vi "Unibot.vi"() -> ()   [LabVIEW 2012]
doc: "Pendubot (Pendulum Robot) consists of a DC motor connected to a link physical rigid link (called here 'elbow\") which is connected to a second rigid link ('arm\") that has no actuation (free spinning link).\n\nThe control objective is to keep the free link in the vertical position while you can choose to balance the controller link (called here elbow) in the extended position (both links are up) or in the contracted position (elbow pointing down and free link up). In those operating points, a State Feedback Control is used to keep in Up-Up or Down-Up position.\n\nThis VI demonstrates how to use Linearization, design of LQR and pole placement controllers and use on swiching controller."
uses:
  <vilib>/Simulation/Scripting/Companion Diagram/SimConfigNode/SimDog.xnode
  <vilib>/Simulation/SignalDisplay/Implementation/NILVSim Time Waveform.llb/SIM Time Waveform (scalar).vi
  <vilib>/Simulation/Implementation/Shared/SIMSCR Execution Mode.ctl
  <vilib>/addons/Control Design/_State Feedback Control/NI_CD_State Feedback Control.lvlib
  <vilib>/addons/Control Design/_Utility/NI_CD_Model Viewer.lvlib
  <vilib>/Simulation/Utility/Implementation/SIM Halt.vi
  Control Systems/Non-linear/Unibot - State Machine Controller.vi
  <vilib>/addons/Control Design/_State Feedback Control/State Feedback Control.llb/State Feedback Control SubVis/cd_Discretized Linear Quadratic Regulator.vi
  <vilib>/Simulation/Scripting/Companion Diagram/SimConfigNode/_simSolvers.ctl
  <vilib>/Simulation/Scripting/Companion Diagram/SimConfigNode/SimParams.ctl
  <vilib>/addons/Control Design/_Model Reduction/NI_CD_Model Reduction.lvlib
  <vilib>/addons/Control Design/_Time Response Analysis/NI_CD_Time Response.lvlib
  <vilib>/addons/Control Design/_Utility/NI_LinSys_Polynomial Math.lvlib
  <vilib>/addons/Control Design/_Frequency Response Analysis/NI_CD_Frequency Response.lvlib
  <vilib>/addons/Control Design/_Model Conversions/NI_CD_Continuous and Discrete.lvlib
  <vilib>/addons/Control Design/_Dynamic Analysis/NI_CD_Dynamic Analysis.lvlib
  <vilib>/Simulation/Implementation/XNodeFramework/SimXNode/SimX.xnode
  <vilib>/Platform/TimedLoop/XDataNode/wakeup.ctl
  <vilib>/Platform/TimedLoop/XDataNode/XDNodeRunTimeDep.lvlib
  <vilib>/Platform/TimedLoop/XDataNode/nitl_modes.ctl
  <vilib>/Platform/TimedLoop/XDataNode/timing_clust.ctl
  <vilib>/Platform/TimedLoop/XDataNode/XDataNode.xnode
  <vilib>/addons/Control Design/_Model Conversions/Continuous and Discrete.llb/Continuous and Discrete SubVI/cd_Convert Continuous to Discrete (SS).vi
  <vilib>/addons/Control Design/_Model Reduction/Model Reduction.llb/Model Reduction SubVIs/cd_Remove I-O-S from SS Model.vi
  <vilib>/addons/Control Design/_Time Response Analysis/Time Response.llb/Time Response subVI/cd_Impulse Response (State-Space).vi
  <vilib>/addons/Control Design/_Time Response Analysis/Time Response.llb/Time Response subVI/cd_Parametric Time Response (SS with External Response).vi
  <vilib>/addons/Control Design/_Frequency Response Analysis/Frequency Response.llb/Frequency Response subVI/cd_Bode (State Space).vi
  <vilib>/addons/Control Design/_Dynamic Analysis/Dynamic Analysis.llb/Dynamic Analysis subVI/cd_Pole-Zero Map (State-Space).vi
  <vilib>/addons/Control Design/_Dynamic Analysis/Dynamic Analysis.llb/Dynamic Analysis subVI/cd_Stability (State-Space).vi
  <vilib>/addons/Control Design/_Utility/Model Viewer.llb/Model Viewer SubVI/cd_Draw State-Space Equation (SS).vi
  <vilib>/addons/Control Design/_State Feedback Control/State Feedback Control.llb/CD State Regulator.vi
  <vilib>/Simulation/Implementation/Shared/SIM Bundle Sim Info.vi
  <vilib>/Simulation/Implementation/Shared/SIM Unbundle Sim Info.vi
  <vilib>/Simulation/Implementation/Shared/NILVSim_FinalizeModel.vi
  <vilib>/Simulation/Implementation/Shared/NILVSim_GetModelError.vi
  <vilib>/Simulation/Implementation/Shared/NILVSim_Initialize.vi
  <vilib>/Simulation/Implementation/Shared/NILVSim_FinishedLate.vi
  <vilib>/Simulation/Utility/Implementation/NILVSim Get Time and IsAcceptedStep.vi
  <vilib>/Simulation/Implementation/Shared/NILVSim_Manager.vi
  <vilib>/Simulation/Implementation/Shared/NI_SIM_Implementation.lvlib
  <vilib>/Simulation/Param Hierarchy/Typedefs/SIMPH Param Control Actions.ctl
  <vilib>/Simulation/Implementation/Shared/NILVSim_ParamChanged.vi
  <vilib>/Utility/error.llb/Clear Errors.vi
  <vilib>/Simulation/Implementation/Shared/SIMSH Read Queue.vi
  <vilib>/Simulation/Utility/Implementation/NILVSim Memory.llb/NILVSim Memory (core).vi
  <vilib>/Simulation/Implementation/Shared/SIM Fire Discrete SubVI.vi
  <vilib>/Simulation/Scripting/Editor Utilities/SIM subVI execution type.ctl
  <vilib>/Simulation/Scripting/Editor Utilities/SIM subVI tag data.ctl
  <vilib>/addons/Control Design/_Model Construction/Model Typedefs.llb/CD General Elements.ctl
  <vilib>/addons/Control Design/_Model Construction/NI_LinSys_Model Typedefs.lvlib
  <vilib>/addons/Control Design/_Model Construction/Model Typedefs.llb/CD State Space Model (MIMO).ctl
panel:
  in  "IMU Pitch":i32(slide) scale=-450.0..450.0
  in  "IMU Roll":i32(slide) scale=-450.0..450.0
  in  "IMU VISA":refnum<visa-resource-name>="COM5"
  out "Received Array":u8[](array[numeric]) format="%02x"
  out "Processing Loop Count":i32
  out "Received array Size":i32
  out "YAW":dbl(knob) scale=-180.0..180.0
  out "Read Loop Count":i32
  out "Serial Settings:Number of Bytes at Serial Port":u32
  out "error out":errorcluster
  out "timed out?":bool
  in  "Motor2 Effort":i32(slide) scale=-450.0..450.0
  in  "Motor1 Effort":i32(slide) scale=-450.0..450.0
  out "Command to Serial":string
  in  "stop?":bool
  out "result":bool
  out "Byte Count":u32
  out "Error Out":errorcluster
  in  "Error In":errorcluster
  out "Gain":dbl[][](array[numeric])=[[13.362365480735772, 19.05380394095224, 1.2104119144158012, 2.4013527998190582]]
  out "State-Space Model":T1={"properties"={"Model name"="", "Input names"=["Torque (Tau)"], "Output names"=["theta1", "theta2"], "Input Delays"=[0.0], "Output Delays"=[0.0, 0.0], "Sampling Time"=0.0, "Notes"=""}, "A"=[[0.0, 0.0, 1.0, 0.0], [0.0, 0.0, 0.0, 1.0], [-54.92473360770753, 40.408778283769514, -1.4920114239882594, 7.105427357601002e-15], [45.63201235945519, 58.19855210917706, 1.492011423988302, -0.22573956409963358]], "B"=[[0.0], [0.0], [29.84022847976503], [3.9334375679108007]], "C"=[[1.0, 0.0, 0.0, 0.0], [0.0, 0.9999999998433566, 0.0, 0.0]], "D"=[[0.0], [0.0]], "StateNames"=["/teta1", "/teta2", "/dteta1", "/dteta2"], "Transport Delay"=[[0.0], [0.0]]} {"Transport Delay" format="%.2f"; "D" format="%#.2g"; "C" format="%#.2g"; "B" format="%#.2g"; "A" format="%#.2g"; "properties"."Sampling Time" format="%#.6p"; "properties"."Output Delays" format="%.4f"; "properties"."Input Delays" format="%.4f"}
  in  "PD Gains":T3={"Kp Up"=16.55, "Kd Up"=5.1567, "Kp Down"=10.2, "Kd Down"=0.974}
  in  "Tab Control":T4(tab)
  in  "Control Technique":T5(tab)
  in  "Q":dbl[][](array[numeric])=[[10.0, 0.0, 0.0, 0.0], [0.0, 10.0, 0.0, 0.0], [0.0, 0.0, 100.0, 0.0], [0.0, 0.0, 0.0, 1.0]] format="%.2f"
  in  "R":dbl[][](array[numeric])=[[50.0]] format="%.2f"
  in  "Desired Pole Location":cdb[](array[numeric])=[0.8275428216771237+0.0i, 0.9068860314786581+0.0i, 0.9511525717602396+0.0i, 0.9425028249515996+0.0i] format="%.2f"
  out "Optimal Gain \nDown-Up":dbl[](array[numeric])=[13.362365480735772, 19.05380394095224, 1.2104119144158012, 2.4013527998190582] format="%.2f"
  out "Optimal Gain\nDown-Down":dbl[](array[numeric])=[-0.14906178101626644, 0.17686358569380023, 1.1761652926773682, -0.039275718443801] format="%.2f"
  out "Optimal Gain \nUp-Up":dbl[](array[numeric])=[-16.081278889113918, -16.397482495141958, -3.1902773104017657, -2.0364914176335533] format="%.2f"
  in  "Type of Control":bool=TRUE
  out "Linearized Equation for Operating Point":picture
  out "Poles locations":cdb[](array[numeric])=[0.6612119646152013+0.0i, 0.9743397418352502+0.0i, 0.9379855295915182+0.0i, 0.9275584671894643+0.0i] format="%.2f"
  out "Impulse Response":cluster{"time":dbl[], dbl[]}[](graph)
  out "Settling Time 1":dbl=2.363776391897807
  out "Settling Time 2":dbl=2.488531257025747
  out "Bode Magnitude":cluster{"W":dbl[], "Magnitude":dbl[]}[](graph)
  out "Bode Phase":cluster{"W":dbl[], "Magnitude":dbl[]}[](graph)
  out "Pole-Zero Map":cluster{dbl[], dbl[]}[](graph)=[{[-30.459733943866535, -2.5043848732190277, -7.159085784207853, -7.159085784207853], [0.0, 0.0, 0.6196593444828095, -0.6196593444828095]}, {[], []}] caption="Closed Loop System Poles"
  out "Stability":T6(ring)
  out "Zeros":cdb[](array[numeric]) format="%.4f"
  out "Poles":cdb[](array[numeric])=[-30.459733943866535+0.0i, -2.5043848732190277+0.0i, -7.159085784207853+0.6196593444828095i, -7.159085784207853-0.6196593444828095i] format="%.4f"
  out "roll":waveform(dbl)(graph)={"t0"=timestamp(0 s since 1904-01-01), "dt"=1.0, "Y"=[12.566370614359172]}
  out "pitch":waveform(dbl)(graph)={"t0"=timestamp(0 s since 1904-01-01), "dt"=1.0, "Y"=[0.0]}
  out "torque":waveform(dbl)(graph)={"t0"=timestamp(0 s since 1904-01-01), "dt"=1.0, "Y"=[0.0]}
  in  "Halt?":bool
  out "Switching State":string="Bringing home"
  in  "Setpoint":dbl(knob) step=0.01 scale=-0.1..0.1
  # "Pendubot - two link Pendulum with \"elbow\" control"
  # "Objective:"
  # "Pendubot (Pendulum Robot) consists of a DC motor connected to a link physical rigid link (called here 'elbow\") which is connected to a second rigid link ('arm\") that has no actuation (free spinning link).\nThe control objective is to keep the free link in the vertical position while you can choose to balance the controller link (called here elbow) in the extended position (both links are up) or in the contracted position (elbow pointing down and free link up). In those operating points, a State Feedback Control is used to keep in Up-Up or Down-Up position. You can tune those controllers in the Design Tab. The controller also can switch between Down-Down position to any other using state machine to apply another control laws to get to the desired location. The technique used for this operation is called partial feedback linearization and PD controllers were used to implement this system. This example also uses a state-machine to switch between states. To avoid chaotic fall of the pendulum if it can't reach the position, another controller is used to drive the elbow to the stationary position (elbow and free link pointing down)."
  # "Variables:\nTorque (Tau): Voltage applied controller\nTheta1: Encoder Position of the controlled link*\nTheta2: Encoder Position of the free link*\n\n*Enconders have zero reference point down"
  # "Up-Up Position"
  # "Down-Down Position"
  # "Down-Up Position"
  # "In this position, the\nelbow is pointing down and free link is controlled in the up position."
  # "In this position, the elbow and free link are pointing down. This is also a stable position and simulation starts from this point."
  # "In this position, the\nelbow and free link is controlled in the up position, similar to an inverted pendulum."
  # "Description:"
  # "The allow the system of such complex machine, we need to develop control techniques based on different states. We have a total of 7 controllers that are controlled by a state-macine that switches whenever the condition is stabilished. The \"down-down\"position is considered to be initial state. Whenever the system doesn't meet specific command, the state machine will bring the system to the down-down position. This controller is designed using a Linear Quadratic Regulator with the model linearized at the down-down position. \n\nTo transition between the Down-Down position to Down-Up and Up-Up position, it is used a nonlinear control technique called \"Feedback Linearization\". The implementation of the controller is using a Proportional-Derivative (PD) controller, which is tuned by 'experimentation' in this case.\n\nThe same LQR technique is applied to obtain the controller around the Up-Up and the Down-Up position.  The gain are designed in the 'Control Design' tab and your objective is to choose the gain that makes the controller stable and resistent to disturbance."
  # "State Feedback Controller\nwith state machine"
  # "Initialize"
  # "Swing Up?"
  # "Swing Down?"
  # "Down-Down\nPosition"
  # "Feedback\nlinearization\nPD controller"
  # "Feedback\nlinearization\nPD controller"
  # "Out of\n bounds?"
  # "Out of\n bounds?"
  # "State\nFeedback\nDown-Down"
  # "In bounds?"
  # "In bounds?"
  # "State\nFeedback\nDown-Up"
  # "State\nFeedback\nUp-Up"
  # "Home?"
  # "Home?"
  # "Encoder\nMeasurements\n(Theta1 and Theta 2)"
  # "DC Motor"
  # "State Feedback Controller\nwith state machine"
  # "Swing Up?"
  # "Swing Down?"
  # "Initialize"
  # "Home?"
  # "Home?"
  # "Control Technique"
  # "Desired\nOperating\nPoint"
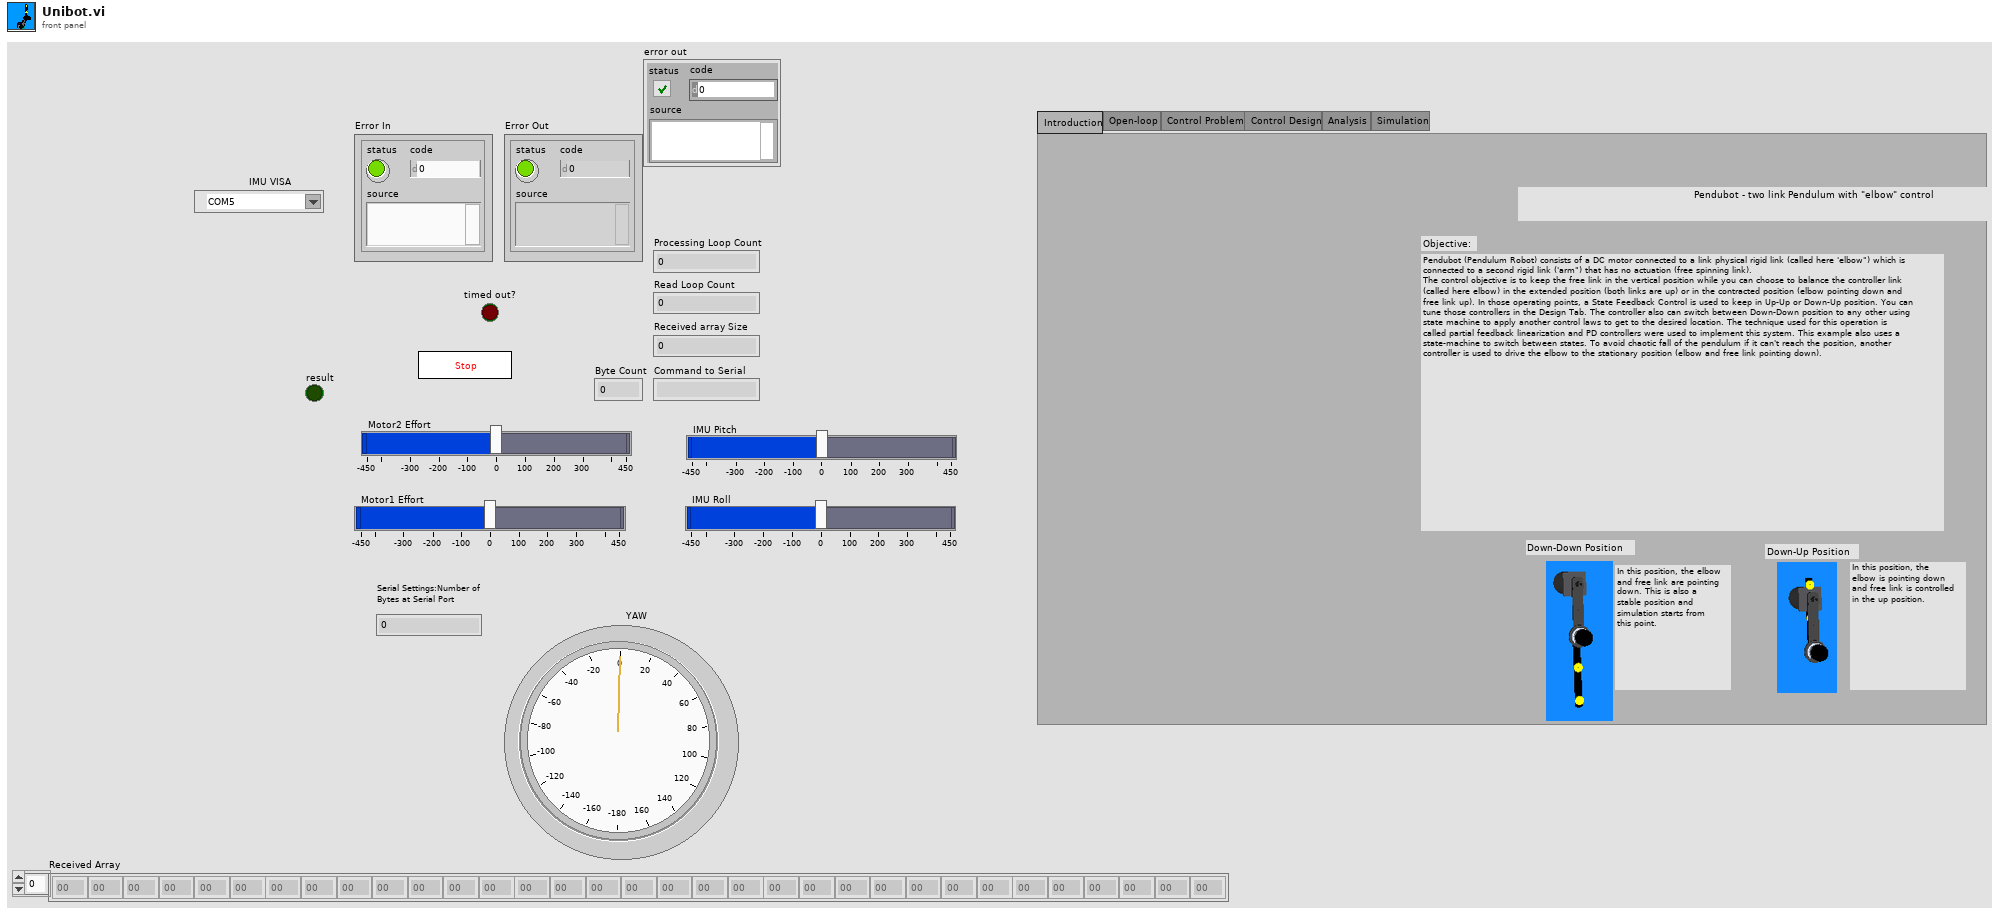
[diagram p1: front panel]
types:
  T1 = typedef "NI_LinSys_Model Typedefs.lvlib/CD State Space Model (MIMO).ctl" = cluster{"properties":T2, "A":dbl[][], "B":dbl[][], "C":dbl[][], "D":dbl[][], "StateNames":string[], "Transport Delay":dbl[][]}
  T2 = typedef "NI_LinSys_Model Typedefs.lvlib/CD General Elements.ctl" = cluster{"Model name":string, "Input names":string[], "Output names":string[], "Input Delays":dbl[], "Output Delays":dbl[], "Sampling Time":dbl, "Notes":string}
  T3 = cluster{"Kp Up":dbl, "Kd Up":dbl, "Kp Down":dbl, "Kd Down":dbl}
  T4 = enum32{"Introduction", "Open-loop", "Control Problem", "Control Design", "Analysis", "Simulation"}
  T5 = enum32{"Linear Quadratic Regulator", "Pole Placement"}
  T6 = enum16{"stable", "marginally stable", "unstable", "undetermined"}
  T7 = enum16{"System Included", "System Included with Noise", "Standalone"}
  T8 = typedef "SIMSCR Execution Mode.ctl" = enum16{"Simulate to Completion", "Single Time-Step Simulation (Fixed Step Only)"}
  T9 = typedef "XDNodeRunTimeDep.lvlib/timing_clust.ctl" = cluster{"Expected End [f-1]":u64, "Actual End [f-1]":u64, "Finished Late? [f-1]":bool, "Expected End [i-1]":u64, "Actual End [i-1]":u64, "Finished Late? [i-1]":bool, "Expected Start [i]":u64, "Actual Start [i]":u64, "Expected Start [f]":u64, "Actual Start [f]":u64, "Source Name":string, "Structure Name":string, "Period":i64, "Deadline":i64, "Offset":i64, "Start":i64, "Priority":i32, "Timeout":i32, "Mode":T10, "Wakeup Reason":T11, "Error":errorcluster, "Source Type":string, "Secondary Source Type":string, "Global End Time":u64, "Global Start Time":u64, "Frame Duration":u64, "Iteration Duration":u64, "Assigned CPU":i32, "I/O Scan Engine Mode":u32}
  T10 = typedef "XDNodeRunTimeDep.lvlib/nitl_modes.ctl" = enum32{"No Change", "Process missed periods, maintain original phase", "Discard missed periods, maintain original phase", "Process missed periods, ignore original phase", "Discard missed periods, ignore original phase"}
  T11 = typedef "XDNodeRunTimeDep.lvlib/wakeup.ctl" = enum32{"Normal", "Aborted", "Asynchronous wakeup", "Timing source error", "Timed loop error", "Timeout"}
  T12 = typedef "SIMPH Param Control Actions.ctl" = enum16{"get params", "set params"}
  T13 = typedef "SIM subVI tag data.ctl" = cluster{"period":dbl, "skew":dbl, "Simulation execution type":T14}
  T14 = typedef "SIM subVI execution type.ctl" = enum16{"Function call", "Discrete", "Continuous", "Initialization only", "Final step only"}
  T15 = typedef "SimParams.ctl" = cluster{"Initial Time (s)":dbl, "Final Time (s)":dbl, "Step Size (s)":dbl, "ODE Solver":T16, "Minimum Step Size (s)":dbl, "Maximum Step Size (s)":dbl, "Relative Tolerance":dbl, "Absolute Tolerance":dbl, "Software Timing":bool, "Initial Step Size (s)":dbl, "Automatic Fixed Step Size?":bool, "Automatic Discrete Step Size?":bool, "Discrete Step Size (s)":dbl, "Calculate using Time Step":bool, "Solver Wired?":bool, "Prev.Frm.Expected End":u64, "Prev.Frm.Actual End":u64, "Prev.Frm.Finished Late?":bool, "Prev.Iter.Expected End":u64, "Prev.Iter.Actual End":u64, "Prev.Iter.Finished Late?":bool, "Expected Iteration Start":u64, "Actual Iteration Start":u64, "Expected Frame Start":u64, "Actual Frame Start":u64, "Source Name":string, "Name":string, "Period":i64, "Deadline":i64, "Offset":i64, "Start":i64, "Priority":i32, "Timeout":i32, "Processor":i32, "Mode":enum32{"No Change", "Process missed periods, maintain original phase", "Discard missed periods, maintain original phase", "Process missed periods, ignore original phase", "Discard missed periods, ignore original phase"}, "Wakeup reason":enum32{"Normal", "Aborted", "Asynchronous wakeup", "Timing source error", "Timed loop error", "Timeout"}, "Error":errorcluster, "Source Type":string, "Secondary Source Type":string, "Global End Time":u64, "Global Start Time":u64, "Full Solver Reset":bool, "Execution Mode":T8, "Nan/Inf Check":bool, "Custom Solver Library":string, "Solver Is Variable":bool, "custom solver name":string, "Signal Collection Decimation":u32}
  T16 = typedef "_simSolvers.ctl" = enum16{"Runge-Kutta 1 (Euler)", "Runge-Kutta 2", "Runge-Kutta 3", "Runge-Kutta 4", "Runge-Kutta 23 (variable)", "Runge-Kutta 45 (variable)", "BDF (variable)", "Adams-Moulton (variable)", "Rosenbrock (variable)", "Discrete States Only", "SDIRK 4 (variable)", "Radau 5 (variable)", "Radau 9 (variable)", "Radau 13 (variable)", "Radau [Variable Order] (variable)", "Gear's Method (variable)", "Linearizer", "State Query", "Trim Eval", "Custom Solver"}
  T17 = typedef "NI_LinSys_Data Typedefs.lvlib/CD MIMO Time Response Data.ctl" = cluster{"Time":dbl[], "Outputs Data":dbl[][][], "States Data":dbl[][][], "plot type":T18}
  T18 = typedef "NI_LinSys_Data Typedefs.lvlib/CD Plot Types Enum.ctl" = enum16{"bode-magnitude", "bode-phase", "nichols", "nyquist", "singular values", "step", "impulse", "initial", "simulation", "nyquist with separation"}
  T19 = typedef "NI_LinSys_Data Typedefs.lvlib/CD Parametric Time Response Data.ctl" = cluster{"Rise Time (s)":dbl[][], "Peak Time (s)":dbl[][], "Settling Time (s)":dbl[][], "Overshoot (%)":dbl[][], "Steady-State Gain":dbl[][], "Peak Value":dbl[][]}
  T20 = typedef "901x DMA FPGA Reference.ctl" = refnum<k20>
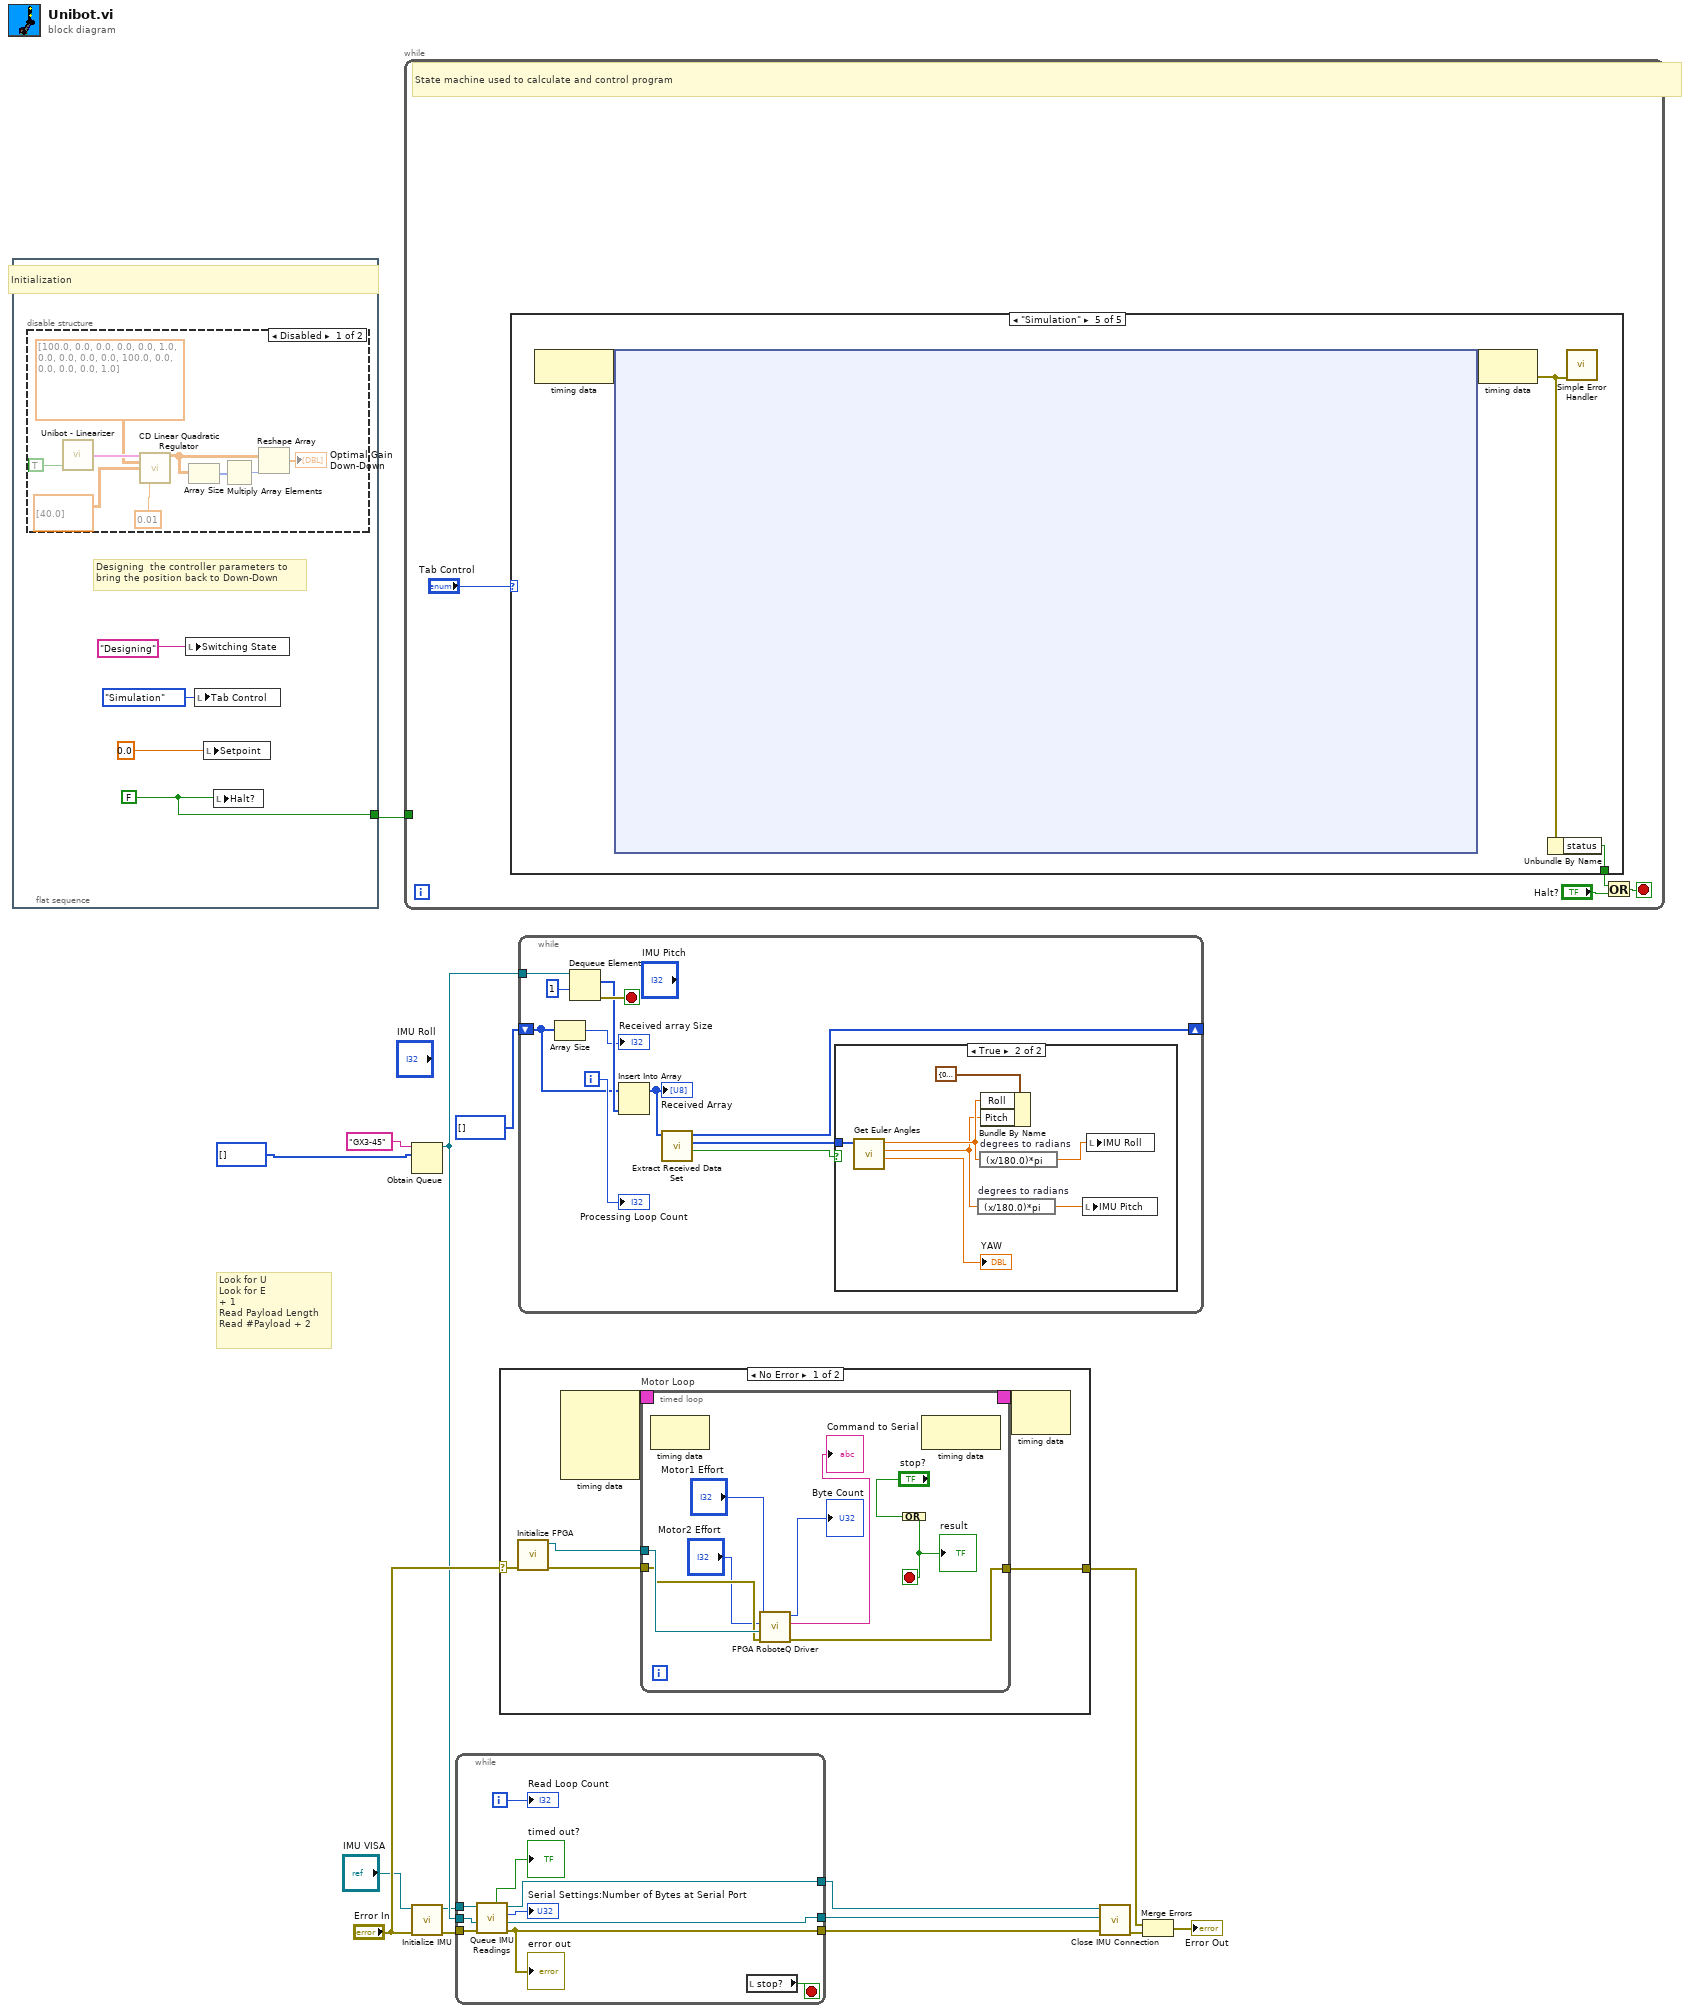
[diagram p0: block diagram]
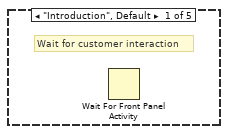
[diagram p5: hidden frame]
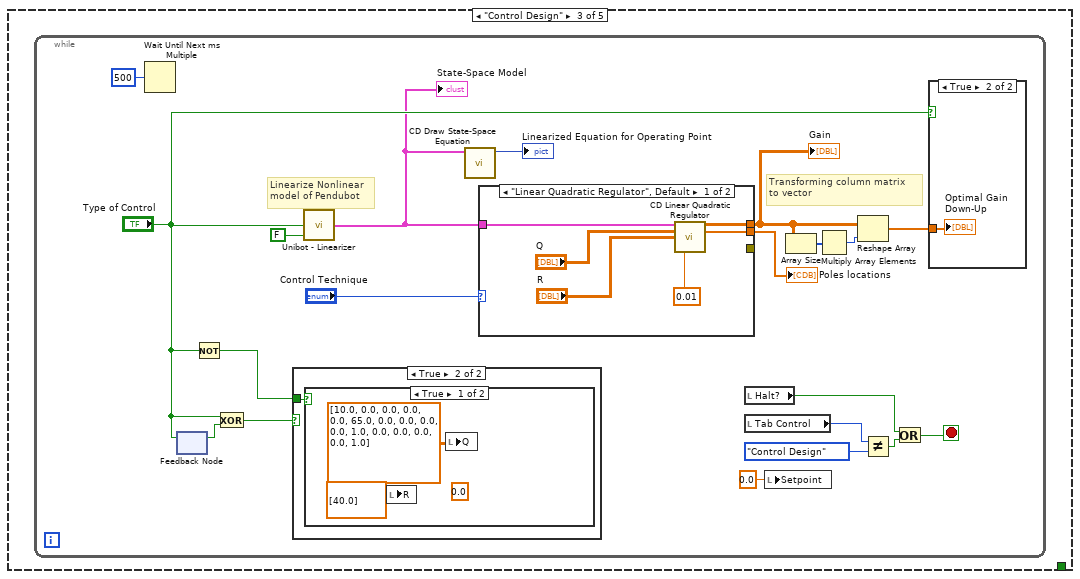
[diagram p7: hidden frame]
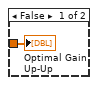
[diagram p8: hidden frame]
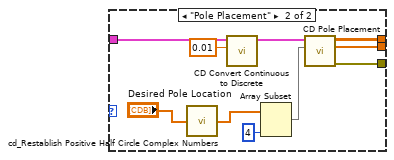
[diagram p9: hidden frame]
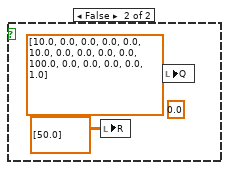
[diagram p11: hidden frame]
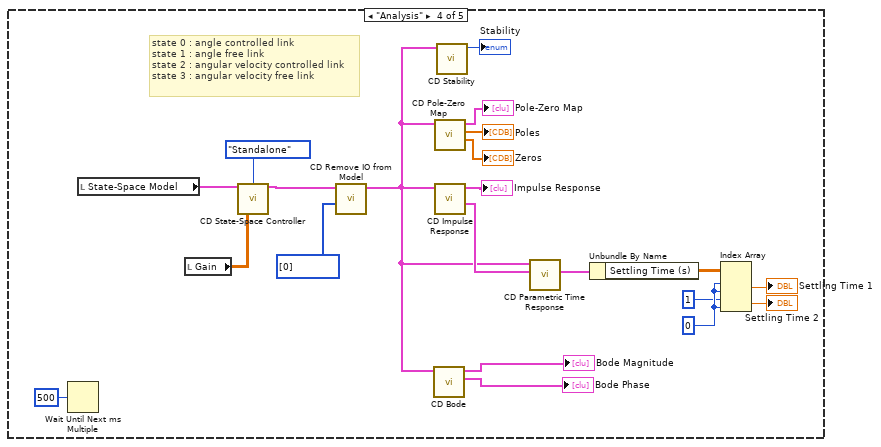
[diagram p12: hidden frame]
diagram:
  # "Look for U\nLook for E\n+ 1\nRead Payload Length\nRead #Payload + 2"
  n1 = flat-sequence {
    tunnel: [w18] -> w15
    frame #0 {
      w18 = FALSE ("Halt?")
      # "Designing  the controller parameters to \nbring the position back to Down-Down"
      # "Initialization"
      n2 = disable-structure shown="Disabled" {
        frame Disabled {
          n3 = call "Unibot - Linearizer.vi"("Down-Down"=TRUE) -> ("State-Space Model"=w27:T1)  [unwired: 1 in, 3 out]
          n4 = call-poly <vilib>:"CD Linear Quadratic Regulator.vi"("Continuous State-Space Model"=w27, "Q"=dbl[][] [[100.0, 0.0, 0.0, 0.0], [0.0, 1.0, 0.0, 0.0], [0.0, 0.0, 100.0, 0.0], [0.0, 0.0, 0.0, 1.0]], "R"=dbl[][] [[40.0]], "Sampling Time (s)"=0.01) -> ("Optimal Gain (K)"=w24:dbl[][])  [unwired: 2 in, 9 out]
          n5 = Array Size(array=w24) -> (size(s)=w26:i32[])
          n6 = Multiply Array Elements(1:w26) -> (0:w25:i32)
          n7 = Reshape Array(w24, w25) -> (→"Optimal Gain\nDown-Down":dbl[])
        }
        frame Enabled {
        }
      }
      n8 = local write "Switching State"("Designing" ("Switching State")) -> ()
      n9 = local write "Tab Control"(T4."Simulation" ("Tab Control")) -> ()
      n10 = local write "Setpoint"(0.0 ("Setpoint")) -> ()
      n11 = local write "Halt?"(w18) -> ()
    }
  }
  n12 = while {
    tunnel: w15 -> [_]
    stop <- w30 stop-if-true
    # "State machine used to calculate and control program"
    n13 = case shown="\"Simulation\"" "Tab Control" {
      tunnel: [_ _ _ _ w97] -> w29
      frame "Introduction", Default {
        # "Wait for customer interaction"
        n14 = Wait For Front Panel Activity() -> ()  [unwired: 3 in, 1 out]
      }
      frame "Open-loop" {
      }
      frame "Control Design" {
        n15 = while {
          stop <- w44 stop-if-true
          # "Linearize Nonlinear\nmodel of Pendubot"
          # "Transforming column matrix\nto vector"
          n16 = Wait Until Next ms Multiple(millisecond multiple=u32 500) -> ()  [unwired: 1 out]
          n17 = feedback-in #1("Type of Control") -> ()
          n18 = feedback #1() -> (w50:bool)  [unwired: 1 out]
          n19 = Not(x="Type of Control") -> (.not. x?=w48:bool)
          n20 = Exclusive Or(1:w50, 2:"Type of Control") -> (0:w49:bool)
          n21 = case shown="True" w49 {
            tunnel: w48 -> [_ w71]
            frame False {
            }
            frame True {
              n22 = case shown="True" w71 {
                frame True {
                  (unwired) 0.0 ("initial teta2")
                  n23 = local write "R"(dbl[][] [[40.0]] ("R")) -> ()
                  n24 = local write "Q"(dbl[][] [[10.0, 0.0, 0.0, 0.0], [0.0, 65.0, 0.0, 0.0], [0.0, 0.0, 1.0, 0.0], [0.0, 0.0, 0.0, 1.0]] ("Q")) -> ()
                }
                frame False {
                  (unwired) 0.0 ("initial teta1")
                  n25 = local write "R"(dbl[][] [[50.0]] ("R")) -> ()
                  n26 = local write "Q"(dbl[][] [[10.0, 0.0, 0.0, 0.0], [0.0, 10.0, 0.0, 0.0], [0.0, 0.0, 100.0, 0.0], [0.0, 0.0, 0.0, 1.0]] ("Q")) -> ()
                }
              }
            }
          }
          n27 = call "Unibot - Linearizer.vi"("Type of Control"="Type of Control", "Down-Down"=FALSE) -> ("State-Space Model"=w35:T1)  [unwired: 3 out]
          "State-Space Model" <- w35
          n28 = call-poly <vilib>:"CD Draw State-Space Equation.vi"("State-Space Model"=w35) -> ("Equation"=→"Linearized Equation for Operating Point":picture)  [unwired: 4 in, 6 out]
          n29 = case shown="\"Linear Quadratic Regulator\", Default" "Control Technique" {
            tunnel: [w60 w70] -> w36
            tunnel: w35 -> [w59 w66]
            tunnel: [w56 w69] -> w42
            tunnel: [_ w67] -> _
            frame "Linear Quadratic Regulator", Default {
              n30 = call-poly <vilib>:"CD Linear Quadratic Regulator.vi"("Continuous State-Space Model"=w59, "Q"="Q", "R"="R", "Sampling Time (s)"=0.01) -> ("Optimal Gain (K)"=w60:dbl[][], "Eigenvalues"=w56:cdb[])  [unwired: 2 in, 8 out]
            }
            frame "Pole Placement" {
              n31 = call <vilib>:"cd_Restablish Positive Half Circle Complex Numbers.vi"("Sorted Complex Numbers (Positive Only)"="Desired Pole Location") -> ("Complete Roots"=w63:cdb[])  [unwired: 8 out]
              n32 = call-poly <vilib>:"CD Convert Continuous to Discrete.vi"("Sampling Time (s)"=0.01, "Continuous State-Space Model"=w66) -> ("Discrete State-Space Model"=w65:T1)  [unwired: 7 in, 2 out]
              n33 = Array Subset(array=w63, length=4) -> (w61:cdb[])  [unwired: 1 in]
              n34 = call <vilib>:"CD Pole Placement.vi"("Poles"=w61, "State-Space Model"=w65) -> ("error out"=w67:errorcluster, "Actual Poles"=w69:cdb[], "Gain"=w70:dbl[][])  [unwired: 2 in, 5 out]
            }
          }
          "Poles locations" <- w42
          "Gain" <- w36
          n35 = local read "Halt?"() -> (w45:bool)
          n36 = local read "Tab Control"() -> (w43:T4)
          n37 = local write "Setpoint"(0.0 ("Gauge")) -> ()
          n38 = Array Size(array=w36) -> (size(s)=w52:i32[])
          n39 = Multiply Array Elements(1:w52) -> (0:w51:i32)
          n40 = Reshape Array(w36, w51) -> (w40:dbl[])
          n41 = Not Equal?(x=w43, y=T4."Control Design") -> (x != y?=w46:bool)
          n42 = Or(x=w45, y=w46) -> (x .or. y?=w44:bool)
          n43 = case shown="True" "Type of Control" {
            tunnel: w40 -> [w53 w54]
            frame False {
              "Optimal Gain \nUp-Up" <- w53
            }
            frame True {
              "Optimal Gain \nDown-Up" <- w54
            }
          }
        }
      }
      frame "Analysis" {
        w87 = 0 ("index (row)")
        # "state 0 : angle controlled link\nstate 1 : angle free link\nstate 2 : angular velocity controlled link\nstate 3 : angular velocity free link"
        n44 = Wait Until Next ms Multiple(millisecond multiple=u32 500) -> ()  [unwired: 1 out]
        n45 = local read "State-Space Model"() -> (w95:T1)
        n46 = local read "Gain"() -> (w93:dbl[][])
        n47 = call-poly <vilib>:"CD State-Space Controller.vi"("State-Space Model"=w95, "Configuration"=T7."Standalone", "Controller Gain (K)"=w93) -> ("Controller Model"=w92:T1)  [unwired: 11 in, 1 out]
        n48 = call-poly <vilib>:"CD Remove IO from Model.vi"("State-Space Model"=w92, "Outputs"=i32[] [0]) -> ("Reduced Model"=w80:T1)  [unwired: 7 in, 1 out]
        n49 = call-poly <vilib>:"CD Bode.vi"("State-Space Model"=w80) -> ("Bode Phase"=→"Bode Phase":cluster{"W":dbl[], "Magnitude":dbl[]}[], "Bode Magnitude"=→"Bode Magnitude":cluster{"W":dbl[], "Magnitude":dbl[]}[])  [unwired: 6 in, 3 out]
        n50 = call-poly <vilib>:"CD Pole-Zero Map.vi"("State-Space Model"=w80) -> ("Zeros"=→"Zeros":cdb[], "Poles"=→"Poles":cdb[], "Pole-Zero Map"=→"Pole-Zero Map":cluster{dbl[], dbl[]}[])  [unwired: 7 in, 1 out]
        n51 = call-poly <vilib>:"CD Impulse Response.vi"("State-Space Model"=w80) -> ("Impulse Response Data"=w90:T17, "Impulse Response Graph"=→"Impulse Response":cluster{"time":dbl[], dbl[]}[])  [unwired: 7 in, 2 out]
        n52 = call-poly <vilib>:"CD Stability.vi"("State-Space Model"=w80) -> ("Stability"=→"Stability":T6)  [unwired: 8 in, 2 out]
        n53 = call-poly <vilib>:"CD Parametric Time Response.vi"("Time Response Data"=w90, "State-Space Model"=w80) -> ("Time Response Parametric Data"=w89:T19)  [unwired: 8 in, 1 out]
        n54 = Unbundle By Name(w89) -> ("Settling Time (s)"=w81:dbl[][])
        n55 = Index Array(array=w81, index (row) #1=w87, index (col) #1=w87, index (row) #2=1 ("index (row)"), index (col) #2=w87) -> (element #1=→"Settling Time 1":dbl, element #2=→"Settling Time 2":dbl)
      }
      frame "Simulation" {
        n56 = node-c288() -> (w100:variant)  [unwired: 1 out]
        n57 = node-c254 ("Simulation Loop 2")(w100) -> (w99:variant)
        n58 = node-c288(w99) -> (w98:errorcluster)
        n59 = Unbundle By Name(w98) -> ("status"=w97:bool)
        n60 = call <vilib>:"Simple Error Handler.vi"("error in (no error)"=w98) -> ()  [unwired: 1 in, 8 out]
      }
    }
    n61 = Or(x=w29, y="Halt?") -> (x .or. y?=w30:bool)
  }
  n62 = Obtain Queue(name (unnamed)="GX3-45", element data type=u8[] [] ("unsigned byte array")) -> (queue out=w10:refnum<queue>)  [unwired: 3 in, 2 out]
  n63 = call "Initialize IMU.vi"("error in (no error)"="Error In", "IMU VISA"="IMU VISA") -> ("error out"=w7:errorcluster, "VISA resource name out"=w6:refnum<visa-resource-name>)  [unwired: 8 in]
  n64 = while {
    tunnel: [w514] -> w3
    tunnel: w10 -> [w510]
    tunnel: w7 -> [w517]
    tunnel: w6 -> [w516]
    tunnel: [w512] -> w5
    tunnel: [w511] -> w4
    i -> [w519]
    stop <- w518 stop-if-true
    n65 = call "Queue IMU Readings.vi"("error in (no error)"=w517, "queue"=w510, "reference"=w516) -> ("error out"=w511:errorcluster, "queue out"=w512:refnum<queue>, "Serial Settings:Number of Bytes at Serial Port"=→"Serial Settings:Number of Bytes at Serial Port":u32, "VISA resource name out"=w514:refnum<visa-resource-name>, "timed out?"=→"timed out?":bool)  [unwired: 4 in]
    "error out" <- w511
    n66 = local read "stop?"() -> (w518:bool)
    "Read Loop Count" <- w519
  }
  n67 = case shown="No Error" "Error In" {
    selector: "Error In" -> [w522 w539]
    tunnel: [w523 w539] -> w2
    frame No Error {
      n68 = call "Initialize FPGA.vi"("error in"=w522) -> ("error out"=w521:errorcluster, "FPGA Out"=w520:T20)  [unwired: 9 in]
      n69 = node-c288() -> (w525:T9)  [unwired: 4 in]
      n70 = timed-loop "Motor Loop" {
        timing: w525 -> [_]
        timing-out: [_] -> w524
        tunnel: w520 -> [w532]
        tunnel: w521 -> [w531]
        tunnel: [w526] -> w523
        stop <- w534 stop-if-true
        n71 = node-c288() -> ()  [unwired: 1 in, 1 out]
        n72 = call "FPGA RoboteQ Driver.vi"("error in (no error)"=w531, "FPGA In"=w532, "Motor 2 Effort"="Motor2 Effort", "Motor 1 Effort"="Motor1 Effort") -> ("error out"=w526:errorcluster, "Command to Serial"=→"Command to Serial":string, "Byte Count"=→"Byte Count":u32)  [unwired: 4 in, 1 out]
        n73 = Compound Arithmetic op=OR("stop?") -> (w534:bool)
        "result" <- w534
        n74 = node-c288() -> ()  [unwired: 1 in, 1 out]
      }
      n75 = node-c288(w524) -> ()  [unwired: 1 out]
    }
    frame Error {
    }
  }
  n76 = while {
    tunnel: w10 -> [w550]
    shift-right: [w540] -> _
    shift-left: u8[] [] ("element") -> [w544]
    i -> [w547]
    stop <- w549 stop-if-true
    n77 = Array Size(array=w544) -> (size(s)=→"Received array Size":i32)
    n78 = Dequeue Element(queue=w550, timeout in ms (-1)=1) -> (element=w548:u8[], error out=w549:errorcluster)  [unwired: 1 in, 2 out]
    n79 = Insert Into Array(array=w544, new element=w548) -> (w546:u8[])  [unwired: 1 in]
    "Received Array" <- w546
    n80 = call "Extract Received Data Set.vi"("Received Array In"=w546) -> ("New Data Set Received"=w542:bool, "Extracted Data Set"=w541:u8[], "Received Array Out"=w540:u8[])  [unwired: 7 in, 1 out]
    n81 = case shown="True" w542 {
      tunnel: w541 -> [_ w557]
      frame False {
      }
      frame True {
        n82 = call "Get Euler Angles.vi"("Received Array"=w557) -> ("Yaw (deg)"=→"YAW":dbl, "Pitch (deg)"=w552:dbl, "Roll (deg)"=w554:dbl)  [unwired: 7 in]
        n83 = expression code="(x/180.0)*pi" "degrees to radians"(w552) -> (w551:dbl)
        n84 = expression code="(x/180.0)*pi" "degrees to radians"(w554) -> (w553:dbl)
        n85 = Bundle By Name(cluster=cluster{"Roll":dbl, "Pitch":dbl} {"Roll"=0.0, "Pitch"=0.0} ("Attitude Indicator 2"), "Roll"=w554, "Pitch"=w552) -> ()  [unwired: 1 out]
        n86 = local write "IMU Pitch"(w551) -> ()
        n87 = local write "IMU Roll"(w553) -> ()
      }
    }
    "Processing Loop Count" <- w547
  }
  n88 = call "Close IMU Connection.vi"("Error In"=w4, "queue"=w5, "VISA resource name"=w3) -> ("error out"=w14:errorcluster)  [unwired: 8 in]
  n89 = Merge Errors(w2, w14) -> (→"Error Out":errorcluster)
